vi "ParameterGuess.vi"(8 "error in":errorcluster, 11 "Image IN":T1) -> (0 "error out":errorcluster, 3 "best fit parameters OUT":dbl[](array[numeric]))   [LabVIEW 2015]
uses:
  <vilib>/vision/Image Controls.llb/IMAQ Image.ctl
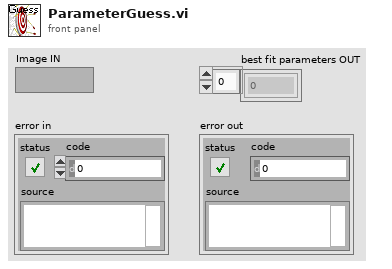
[diagram p1: front panel]
types:
  T1 = typedef "IMAQ Image.ctl" = refnum<image>
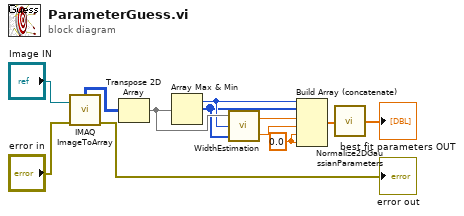
[diagram p0: block diagram]
diagram:
  w6 = 0.0 ("element")
  n1 = call "IMAQ ImageToArray"("error in (no error)"="error in", "Image"="Image IN") -> ("error out"=→"error out":errorcluster, "Image Pixels (U8)"=w1:u8[][])  [unwired: 2 in, 3 out]
  n2 = Transpose 2D Array(2D array=w1) -> (transposed array=w9:u8[][])
  n3 = Array Max & Min(array=w9) -> (max value=w5:u8, max index (indices)=w2:i32[])  [unwired: 2 out]
  n4 = call "WidthEstimation.vi"("maximum index"=w2, "maximium"=w5, "2D Gaussian Data"=w9) -> ("wy Estimated"=w4:dbl, "wx Estimated"=w3:dbl)
  n5 = Build Array (concatenate)(w5, w2, w3, w4, w6, w6) -> (w7:dbl[])
  n6 = call "Normalize2DGaussianParameters.vi"("best fit parameters IN"=w7) -> ("best fit parameters OUT"=→"best fit parameters OUT":dbl[])
